vi "读触点-8位.vi"(8 "error out":errorcluster, 9 "触点类型":string, 10 "读取起始地址":string, 11 "VISA resource name out":refnum<visa-resource-name>) -> (0 "error IO":errorcluster, 1 "通讯延时":u32, 2 "读取布尔数组":bool[](array[boolean]), 3 "VISA resource name out 2":refnum<visa-resource-name>)   [LabVIEW 2018]
uses:
  <vilib>/Instr/_visa.llb/VISA Configure Serial Port (Instr).vi
panel:
  out "子字符串":string
  out "连接的字符串":string
  out "读取缓冲区":string
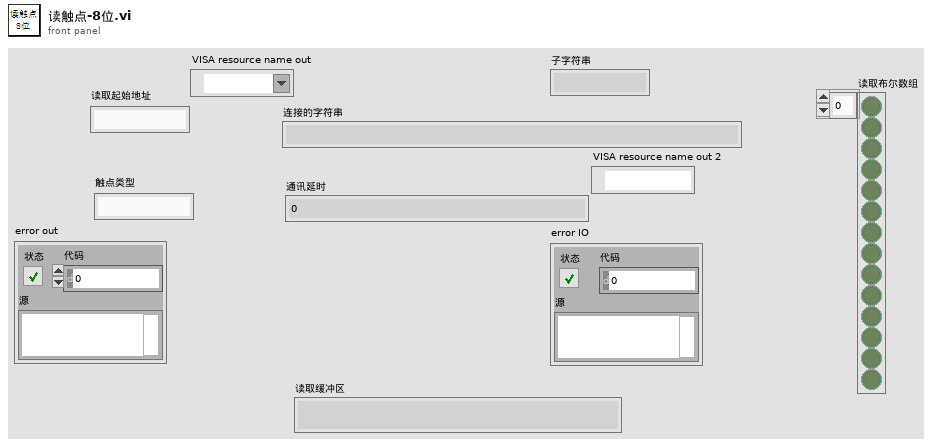
[diagram p1: front panel]
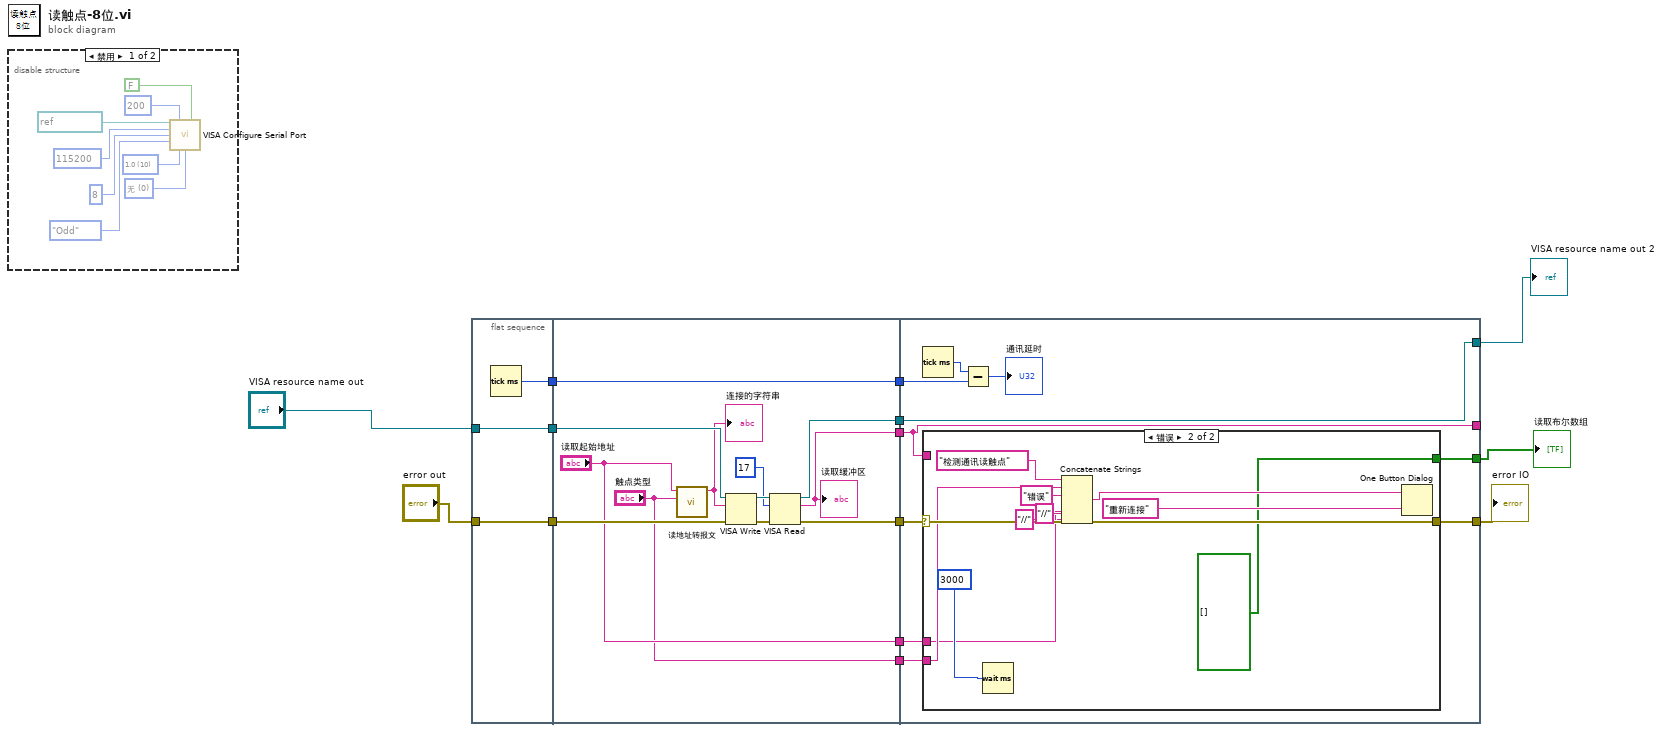
[diagram p0: block diagram]
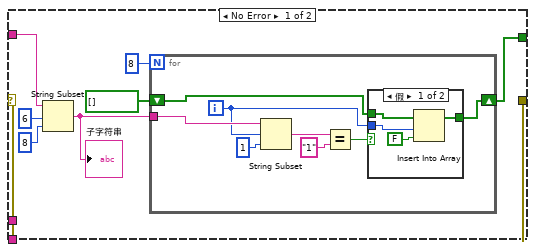
[diagram p3: hidden frame]
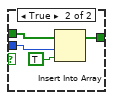
[diagram p4: hidden frame]
diagram:
  n1 = disable-structure shown="禁用" {
    frame Disabled {
      w16 = u16 0 items=["无", "XON/XOFF", "RTS/CTS", "XON/XOFF & RTS/CTS", "DTR/DSR", "XON/XOFF & DTR/DSR"] ("flow control (0:none)")
      w17 = u16 10 items=["1.0"=10, "1.5"=15, "2.0"=20] ("stop bits (10: 1 bit)")
      n2 = call-poly "VISA Configure Serial Port"("VISA resource name"=refnum<visa-resource-name> "COM3", "timeout (10sec)"=u32 200, "Enable Termination\nChar (T)"=FALSE ("Enable Termination\nChar (T)"), "baud rate (9600)"=u32 115200, "data bits (8)"=u16 8, "parity (0:none)"=enum16{"None", "Odd", "Even", "Mark", "Space"}."Odd", "stop bits (10: 1 bit)"=w17, "flow control (0:none)"=w16) -> ()  [unwired: 6 in, 2 out]
    }
    frame Enabled {
    }
  }
  n3 = flat-sequence {
    tunnel: [w25] -> w14
    tunnel: "VISA resource name out" -> [w24]
    tunnel: [w24] -> w13
    tunnel: [w23] -> w12
    tunnel: "error out" -> [w23]
    tunnel: w14 -> [w37]
    tunnel: [w37] -> w11
    tunnel: [w36] -> w10
    tunnel: w13 -> [w35]
    tunnel: w12 -> [w34]
    tunnel: [w32] -> w9
    tunnel: [w28] -> w8
    tunnel: ["读取起始地址"] -> w3
    tunnel: ["触点类型"] -> w2
    tunnel: w11 -> [w46]
    tunnel: w10 -> [w44]
    tunnel: [w43] -> w4
    tunnel: w9 -> [w42]
    tunnel: [w42] -> w5
    tunnel: [w39] -> _
    tunnel: w8 -> [w39]
    tunnel: w3 -> [w41]
    tunnel: w2 -> [w40]
    tunnel: [w38] -> w1
    frame #0 {
      n4 = Tick Count (ms)() -> (millisecond timer value=w25:u32)
    }
    frame #1 {
      n5 = call "读地址转报文.vi"("读取触点类型"="触点类型", "读取起始地址"="读取起始地址") -> ("连接的字符串"=w33:string)  [unwired: 9 in]
      "连接的字符串" <- w33
      n6 = VISA Write(VISA resource name=w35, write buffer=w33, error in (no error)=w34) -> (VISA resource name out=w31:refnum<visa-resource-name>, error out=w30:errorcluster)  [unwired: 1 out]
      n7 = VISA Read(VISA resource name=w31, byte count=u32 17 ("字节总数"), error in (no error)=w30) -> (VISA resource name out=w32:refnum<visa-resource-name>, read buffer=w28:string, error out=w36:errorcluster)  [unwired: 1 out]
      "读取缓冲区" <- w28
    }
    frame #2 {
      n8 = Tick Count (ms)() -> (millisecond timer value=w47:u32)
      n9 = case shown="错误" w44 {
        selector: w44 -> [w55 w82]
        tunnel: [w55 w82] -> w43
        tunnel: w41 -> [_ w75]
        tunnel: w40 -> [_ w78]
        tunnel: w39 -> [w49 _]
        tunnel: [w48 bool[] []] -> w38
        frame No Error {
          n10 = String Subset(string=w49, offset (0)=6 ("偏移量(0)"), length (rest)=8 ("长度（剩余）")) -> (substring=w54:string)
          "子字符串" <- w54
          n11 = for {
            N: 8 -> [_]
            tunnel: w54 -> [w63]
            shift-right: [w56] -> w48
            shift-left: bool[] [] -> [w58]
            i -> [w57]
            n12 = String Subset(string=w63, offset (0)=w57, length (rest)=1 ("长度（剩余）")) -> (substring=w61:string)
            n13 = Equal?(x=w61, y="1") -> (x = y?=w59:bool)
            n14 = case shown="假" w59 {
              tunnel: w58 -> [w67 w71]
              tunnel: w57 -> [w66 w70]
              tunnel: [w64 w68] -> w56
              frame False {
                n15 = Insert Into Array(array=w67, index=w66, new element=FALSE ("新元素/子数组")) -> (w64:bool[])
              }
              frame True {
                n16 = Insert Into Array(array=w71, index=w70, new element=TRUE ("新元素/子数组")) -> (w68:bool[])
              }
            }
          }
        }
        frame Error {
          n17 = Wait (ms)(milliseconds to wait=u32 3000 ("等待时间（毫秒）")) -> ()  [unwired: 1 out]
          n18 = Concatenate Strings("检测通讯读触点" ("消息"), w78, "错误" ("字符串"), "//" ("字符串"), w75, "//" ("字符串")) -> (w73:string)
          n19 = One Button Dialog(message=w73, button name ("OK")="重新连接" ("按钮名称（“确定”）")) -> ()  [unwired: 1 out]
        }
      }
      n20 = Subtract(x=w47, y=w46) -> (x-y=→"通讯延时":u32)
    }
  }
  "读取布尔数组" <- w1
  "VISA resource name out 2" <- w5
  "error IO" <- w4
